vi "Arcade VelociRaptor.vi"(8 "error in (no error)":errorcluster, 9 "Y axis value":dbl, 10 "X axis value":dbl, 11 "RobotDriveDevRef":T1={"DevStatus"={"status"=FALSE, "code"=0, "source"=""}, "Motors[]"=[], "Square Inputs"=FALSE, "Max Output"=1.0}) -> (0 "error out":errorcluster, 2 "Motor Values":dbl[](array[numeric]), 3 "RobotDriveDevRef":T1={"DevStatus"={"status"=FALSE, "code"=0, "source"=""}, "Motors[]"=[], "Square Inputs"=FALSE, "Max Output"=1.0})   [LabVIEW 2014]
doc: "Uses a standard algorithm to configure the motors for arcade driving. This algorithm does not saturate over half of the range.\n\nThis software is licensed. Open the labview\\readme\\WPI Robotics Library Open Source License.txt file for more information."
uses:
  <vilib>/Rock Robotics/WPI/RobotDrive/WPI_RobotDriveDevRef.ctl
  <vilib>/Rock Robotics/WPI/MotorControl/WPI_MotorControlDeviceRef.ctl
  <vilib>/Rock Robotics/WPI/MotorControl/WPI_MotorControlType.ctl
  <vilib>/Rock Robotics/SystemInterfaces/Typedef/FPGA_TypedefDigitalModule.ctl
  <vilib>/Rock Robotics/SystemInterfaces/DIO/FPGA_DIOPWMChannel.ctl
  <vilib>/Rock Robotics/WPI/PWM/WPI_PWMDeadband.ctl
  <vilib>/Rock Robotics/WPI/CAN/Jaguar/SubVIs/WPI_CANJaguar_ControlMode.ctl
  <vilib>/Rock Robotics/WPI/CAN/TalonSRX/WPI_CANTalonSRX_APIControlMode.ctl
  <vilib>/Rock Robotics/WPI/PWM/WPI_PWMTransform_ConPane.ctl
  <vilib>/Rock Robotics/SystemInterfaces/NetworkCommunication/NetComm_UsageReport_ResourceType.ctl
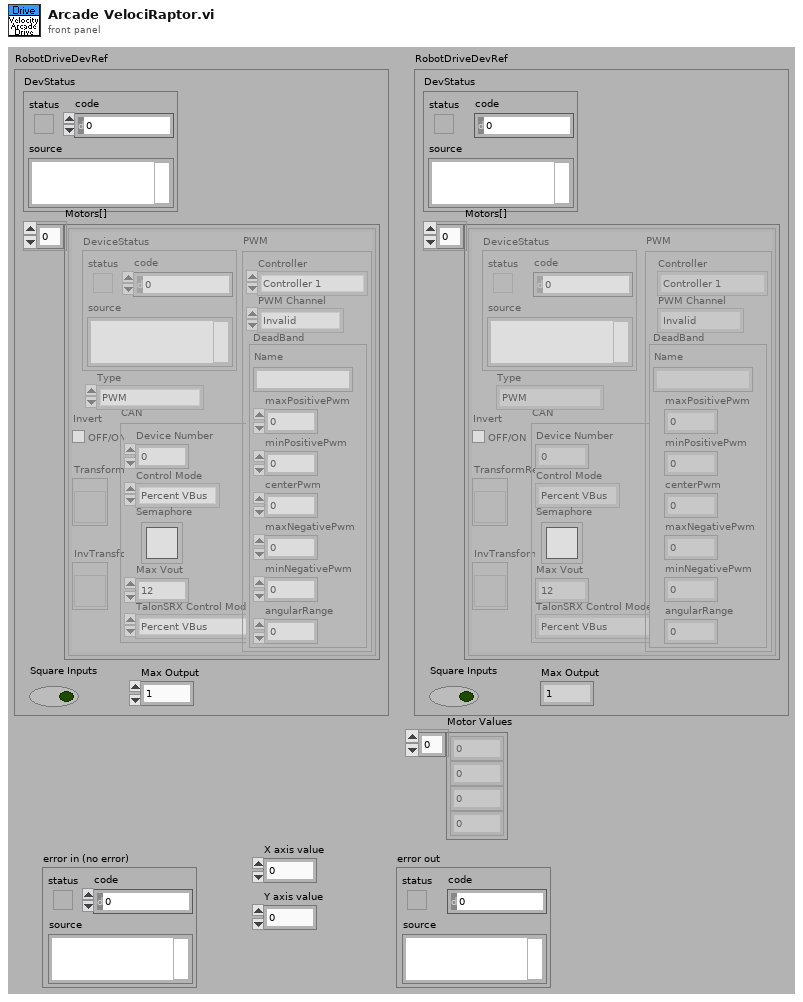
[diagram p1: front panel]
types:
  T1 = typedef "WPI_RobotDriveDevRef.ctl" = cluster{"DevStatus":errorcluster, "Motors[]":T2[], "Square Inputs":bool, "Max Output":dbl}
  T2 = typedef "WPI_MotorControlDeviceRef.ctl" = cluster{"DeviceStatus":errorcluster, "Type":T3, "PWM":cluster{"Controller":T4, "PWM Channel":T5, "DeadBand":T6}, "CAN":cluster{"Device Number":u8, "Control Mode":T7, "Semaphore":T8, "Max Vout":dbl, "TalonSRX Control Mode":T9}, "Invert":bool, "TransformRef":T10, "InvTransformRef":T10}
  T3 = typedef "WPI_MotorControlType.ctl" = enum16{"PWM", "CAN", "CANTalonSRX"}
  T4 = typedef "FPGA_TypedefDigitalModule.ctl" = enum16{"Controller 1"}
  T5 = typedef "FPGA_DIOPWMChannel.ctl" = enum8{"PWM 0", "PWM 1", "PWM 2", "PWM 3", "PWM 4", "PWM 5", "PWM 6", "PWM 7", "PWM 8", "PWM 9", "PWM MXP 0", "PWM MXP 1", "PWM MXP 2", "PWM MXP 3", "PWM MXP 4", "PWM MXP 5", "PWM MXP 6", "PWM MXP 7", "PWM MXP 8", "PWM MXP 9", "Invalid"}
  T6 = typedef "WPI_PWMDeadband.ctl" = cluster{"Name":string, "maxPositivePwm":i32, "minPositivePwm":i32, "centerPwm":i32, "maxNegativePwm":i32, "minNegativePwm":i32, "angularRange":u16}
  T7 = typedef "WPI_CANJaguar_ControlMode.ctl" = enum8{"Percent VBus", "Current", "Speed", "Position", "Voltage"}
  T8 = typedef "Semaphore RefNum" = refnum<k1>
  T9 = typedef "WPI_CANTalonSRX_APIControlMode.ctl" = enum8{"Percent VBus", "Speed", "Position", "Slave", "Unchanged / Invalid"}
  T10 = typedef "WPI_PWMTransform_ConPane.ctl" = refnum<vi>
  T11 = typedef "NetComm_UsageReport_ResourceType.ctl" = enum8{"Controller", "Module", "Language", "CANPlugin", "Accelerometer", "ADXL345", "AnalogChannel", "AnalogTrigger", "AnalogTriggerOutput", "CANJaguar", "Compressor", "Counter", "Dashboard", "DigitalInput", "DigitalOutput", "DriverStationCIO", "DriverStationEIO", "DriverStationLCD", "Encoder", "GearTooth", "Gyro", "I2C", "Framework", "Jaguar", "Joystick", "Kinect", "KinectStick", "PIDController", "Preferences", "PWM", "Relay", "RobotDrive", "SerialPort", "Servo", "Solenoid", "SPI", "Task", "Ultrasonic", "Victor", "Button", "Command", "AxisCamera", "PCVideoServer", "SmartDashboard", "Talon", "HiTechnicColorSensor", "HiTechnicAccel", "HiTechnicCompass", "SRF08", "AnalogOutput", "Victor SP", "Talon SRX", "CAN Talon SRX"}
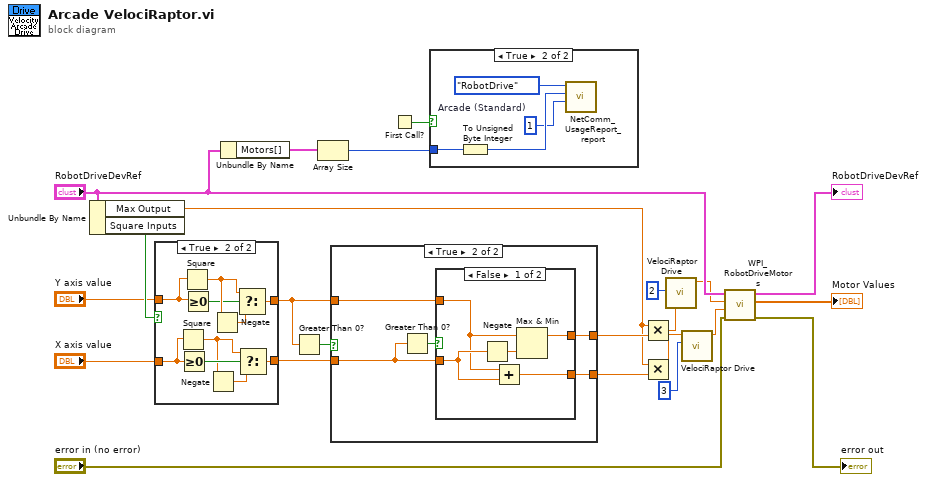
[diagram p0: block diagram]
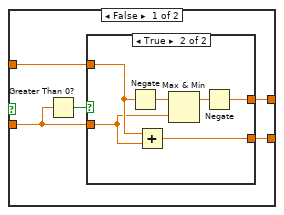
[diagram p3: hidden frame]
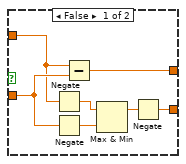
[diagram p4: hidden frame]
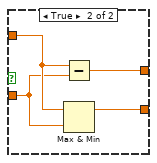
[diagram p5: hidden frame]
diagram:
  n1 = Unbundle By Name("RobotDriveDevRef") -> ("Max Output"=w14:dbl, "Square Inputs"=w22:bool)
  n2 = case shown="True" w22 {
    tunnel: [w24 w35] -> w19
    tunnel: [w25 w34] -> w20
    tunnel: "X axis value" -> [w24 w33]
    tunnel: "Y axis value" -> [w25 w32]
    frame False {
    }
    frame True {
      n3 = Square(x=w33) -> (x^2=w30:dbl)
      n4 = Greater Or Equal To 0?(x=w33) -> (x >= 0?=w31:bool)
      n5 = Square(x=w32) -> (x^2=w27:dbl)
      n6 = Greater Or Equal To 0?(x=w32) -> (x >= 0?=w26:bool)
      n7 = Negate(x=w30) -> (-x=w29:dbl)
      n8 = Negate(x=w27) -> (-x=w28:dbl)
      n9 = Select(t=w27, s=w26, f=w28) -> (s? t:f=w34:dbl)
      n10 = Select(t=w30, s=w31, f=w29) -> (s? t:f=w35:dbl)
    }
  }
  n11 = Unbundle By Name("RobotDriveDevRef") -> ("Motors[]"=w9:T2[])
  n12 = Greater Than 0?(x=w20) -> (x > 0?=w21:bool)
  n13 = Array Size(array=w9) -> (size(s)=w8:i32)
  n14 = case shown="True" w21 {
    tunnel: w19 -> [w39 w57]
    tunnel: w20 -> [w38 w56]
    tunnel: [w37 w55] -> w18
    tunnel: [w36 w54] -> w15
    frame False {
      n15 = Greater Than 0?(x=w39) -> (x > 0?=w40:bool)
      n16 = case shown="True" w40 {
        tunnel: w39 -> [w47 w49]
        tunnel: w38 -> [w45 w50]
        tunnel: [w41 w51] -> w37
        tunnel: [w42 w48] -> w36
        frame False {
          n17 = Negate(x=w45) -> (-x=w46:dbl)
          n18 = Negate(x=w47) -> (-x=w44:dbl)
          n19 = Subtract(x=w45, y=w47) -> (x-y=w41:dbl)
          n20 = Max & Min(x=w46, y=w44) -> (max(x,y)=w43:dbl)  [unwired: 1 out]
          n21 = Negate(x=w43) -> (-x=w42:dbl)
        }
        frame True {
          n22 = Negate(x=w50) -> (-x=w53:dbl)
          n23 = Add(x=w50, y=w49) -> (x+y=w48:dbl)
          n24 = Max & Min(x=w53, y=w49) -> (max(x,y)=w52:dbl)  [unwired: 1 out]
          n25 = Negate(x=w52) -> (-x=w51:dbl)
        }
      }
    }
    frame True {
      n26 = Greater Than 0?(x=w57) -> (x > 0?=w58:bool)
      n27 = case shown="False" w58 {
        tunnel: w57 -> [w63 w65]
        tunnel: w56 -> [w60 w66]
        tunnel: [w61 w64] -> w55
        tunnel: [w59 w67] -> w54
        frame False {
          n28 = Negate(x=w63) -> (-x=w62:dbl)
          n29 = Add(x=w60, y=w63) -> (x+y=w59:dbl)
          n30 = Max & Min(x=w60, y=w62) -> (max(x,y)=w61:dbl)  [unwired: 1 out]
        }
        frame True {
          n31 = Subtract(x=w66, y=w65) -> (x-y=w64:dbl)
          n32 = Max & Min(x=w66, y=w65) -> (max(x,y)=w67:dbl)  [unwired: 1 out]
        }
      }
    }
  }
  n33 = First Call?() -> (First Call?: T/F=w11:bool)
  n34 = case shown="True" w11 {
    tunnel: w8 -> [_ w70]
    frame False {
    }
    frame True {
      w68 = u8 1  # Arcade (Standard)
      n35 = To Unsigned Byte Integer(number=w70) -> (unsigned 8bit integer=w69:u8)
      n36 = call <vilib>:"NetComm_UsageReport_report.vi"("Context"=w68, "Instance Number"=w69, "Resource Type"=NetComm_UsageReport_ResourceType."RobotDrive") -> ()  [unwired: 9 in]
    }
  }
  n37 = Multiply(x=w14, y=w18) -> (x*y=w6:dbl)
  n38 = Multiply(x=w14, y=w15) -> (x*y=w4:dbl)
  n39 = call "VelociRaptor Drive.vi"("Encoder Index"=2, "Throttle in"=w6) -> ("Motor out"=w2:dbl)  [unwired: 9 in]
  n40 = call "VelociRaptor Drive.vi"("Encoder Index"=3, "Throttle in"=w4) -> ("Motor out"=w1:dbl)  [unwired: 9 in]
  n41 = call <vilib>:"WPI_RobotDriveMotors.vi"("error in (no error)"="error in (no error)", "RightSpeed"=w1, "LeftSpeed"=w2, "RobotDriveDevRef"="RobotDriveDevRef") -> ("error out"=→"error out":errorcluster, "Motor Values"=→"Motor Values":dbl[], "RobotDriveDevRef"=→"RobotDriveDevRef":T1)  [unwired: 5 out]
